vi "环境数据发送帧.vi"(10 "环境变量":T1, 11 "用户地址":string) -> (2 "报文长度":i32, 3 "字符串":string)   [LabVIEW 2016, in "环境动力监测库.lvlib" / "NMEA.lvlib"]
uses:
  NMEA.lvlib
panel:
  out "data":T2 {"数据类别" items=["水样数据"=0, "标样数据"=1, "零点核查数据"=2, "跨度核查数据"=3, "环境变量"=4, "水样数据补传"=16, "标样核查数据补传"=17, "零点核查数据补传"=18, "跨度核查数据补传"=19]; "数组"."污染物" items=["水温"=1, "浊度"=2, "DO"=3, "pH"=4, "ORP"=5, "比电导率"=6, "叶绿素a"=7, "氨氮"=8, "亚硝氮"=9, "硫化物"=10, "电压"=11, "温度"=12, "湿度"=13, "GPS经度"=14, "GPS纬度"=15, "BD经度"=16, "BD纬度"=17]; "数组"."标识" items=["N"=1, "T"=2, "L"=3, "D"=4, "Z"=5, "M"=6, "hd"=7]}
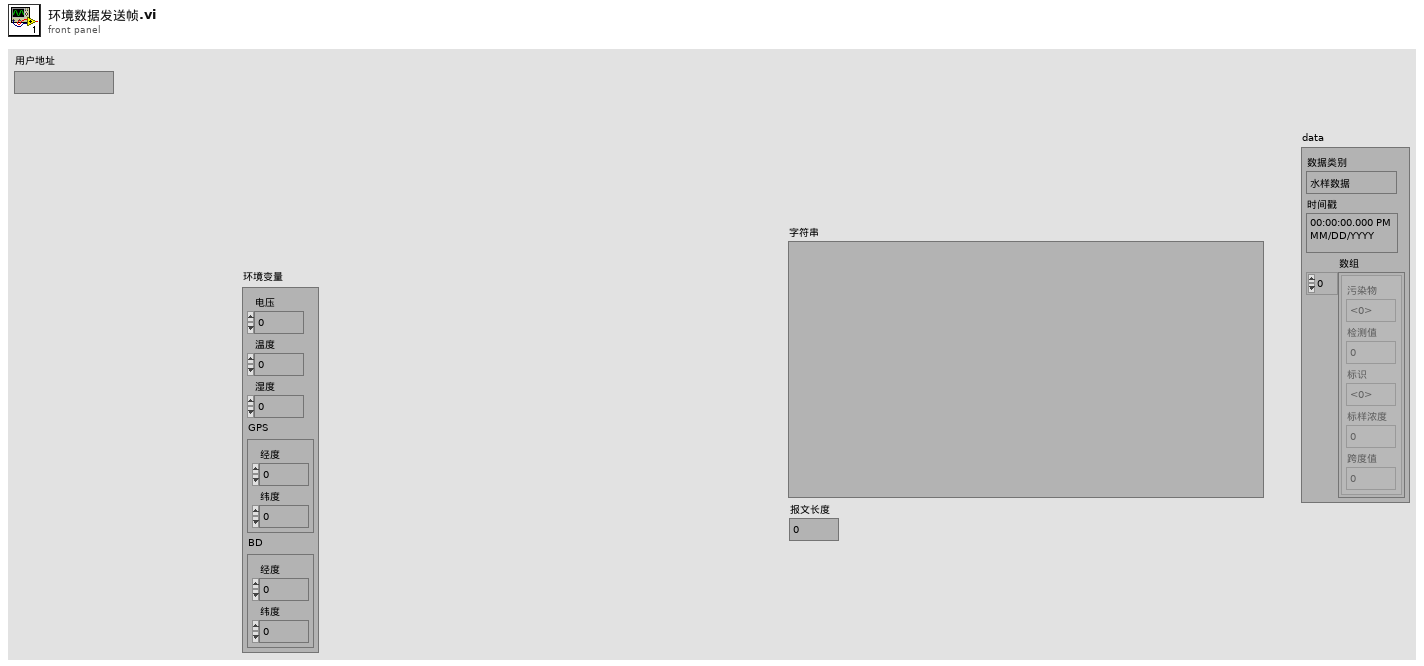
[diagram p1: front panel]
types:
  T1 = cluster{"电压":dbl, "温度":dbl, "湿度":dbl, "GPS":cluster{"经度":dbl, "纬度":dbl}, "BD":cluster{"经度":dbl, "纬度":dbl}}
  T2 = cluster{"数据类别":u16, "时间戳":timestamp, "数组":cluster{"污染物":u16, "检测值":dbl, "标识":u16, "标样浓度":dbl, "跨度值":dbl}[]}
  T3 = cluster{"污染物":u16, "检测值":dbl, "标识":u16, "标样浓度":dbl, "跨度值":dbl}
  T4 = cluster{"污染物":u16, "检测值":dbl, "标识":u16, "标样浓度":dbl, "跨度值":dbl}[]
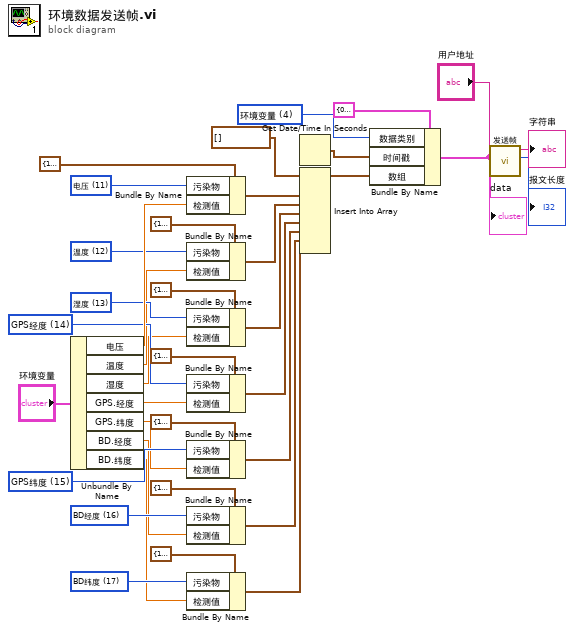
[diagram p0: block diagram]
diagram:
  w14 = u16 17 items=["水温"=1, "浊度"=2, "DO"=3, "pH"=4, "ORP"=5, "比电导率"=6, "叶绿素a"=7, "氨氮"=8, "亚硝氮"=9, "硫化物"=10, "电压"=11, "温度"=12, "湿度"=13, "GPS经度"=14, "GPS纬度"=15, "BD经度"=16, "BD纬度"=17] ("污染物")
  w15 = u16 16 items=["水温"=1, "浊度"=2, "DO"=3, "pH"=4, "ORP"=5, "比电导率"=6, "叶绿素a"=7, "氨氮"=8, "亚硝氮"=9, "硫化物"=10, "电压"=11, "温度"=12, "湿度"=13, "GPS经度"=14, "GPS纬度"=15, "BD经度"=16, "BD纬度"=17] ("污染物")
  w18 = u16 15 items=["水温"=1, "浊度"=2, "DO"=3, "pH"=4, "ORP"=5, "比电导率"=6, "叶绿素a"=7, "氨氮"=8, "亚硝氮"=9, "硫化物"=10, "电压"=11, "温度"=12, "湿度"=13, "GPS经度"=14, "GPS纬度"=15, "BD经度"=16, "BD纬度"=17] ("污染物")
  w19 = u16 14 items=["水温"=1, "浊度"=2, "DO"=3, "pH"=4, "ORP"=5, "比电导率"=6, "叶绿素a"=7, "氨氮"=8, "亚硝氮"=9, "硫化物"=10, "电压"=11, "温度"=12, "湿度"=13, "GPS经度"=14, "GPS纬度"=15, "BD经度"=16, "BD纬度"=17] ("污染物")
  w22 = u16 13 items=["水温"=1, "浊度"=2, "DO"=3, "pH"=4, "ORP"=5, "比电导率"=6, "叶绿素a"=7, "氨氮"=8, "亚硝氮"=9, "硫化物"=10, "电压"=11, "温度"=12, "湿度"=13, "GPS经度"=14, "GPS纬度"=15, "BD经度"=16, "BD纬度"=17] ("污染物")
  w23 = u16 12 items=["水温"=1, "浊度"=2, "DO"=3, "pH"=4, "ORP"=5, "比电导率"=6, "叶绿素a"=7, "氨氮"=8, "亚硝氮"=9, "硫化物"=10, "电压"=11, "温度"=12, "湿度"=13, "GPS经度"=14, "GPS纬度"=15, "BD经度"=16, "BD纬度"=17] ("污染物")
  w26 = u16 11 items=["水温"=1, "浊度"=2, "DO"=3, "pH"=4, "ORP"=5, "比电导率"=6, "叶绿素a"=7, "氨氮"=8, "亚硝氮"=9, "硫化物"=10, "电压"=11, "温度"=12, "湿度"=13, "GPS经度"=14, "GPS纬度"=15, "BD经度"=16, "BD纬度"=17] ("污染物")
  w30 = u16 4 items=["水样数据"=0, "标样数据"=1, "零点核查数据"=2, "跨度核查数据"=3, "环境变量"=4, "水样数据补传"=16, "标样核查数据补传"=17, "零点核查数据补传"=18, "跨度核查数据补传"=19] ("数据类别")
  n1 = Unbundle By Name("环境变量") -> ("电压"=w25:dbl, "温度"=w6:dbl, "湿度"=w5:dbl, "GPS.经度"=w4:dbl, "GPS.纬度"=w3:dbl, "BD.经度"=w2:dbl, "BD.纬度"=w1:dbl)
  n2 = Bundle By Name(cluster=T3 {"污染物"=11, "检测值"=0.0, "标识"=0, "标样浓度"=0.0, "跨度值"=0.0} ("数据"), "污染物"=w26, "检测值"=w25) -> (w34:T3)
  n3 = Bundle By Name(cluster=T3 {"污染物"=11, "检测值"=0.0, "标识"=0, "标样浓度"=0.0, "跨度值"=0.0} ("数据"), "污染物"=w23, "检测值"=w6) -> (w12:T3)
  n4 = Bundle By Name(cluster=T3 {"污染物"=11, "检测值"=0.0, "标识"=0, "标样浓度"=0.0, "跨度值"=0.0} ("数据"), "污染物"=w22, "检测值"=w5) -> (w11:T3)
  n5 = Bundle By Name(cluster=T3 {"污染物"=11, "检测值"=0.0, "标识"=0, "标样浓度"=0.0, "跨度值"=0.0} ("数据"), "污染物"=w19, "检测值"=w4) -> (w10:T3)
  n6 = Bundle By Name(cluster=T3 {"污染物"=11, "检测值"=0.0, "标识"=0, "标样浓度"=0.0, "跨度值"=0.0} ("数据"), "污染物"=w18, "检测值"=w3) -> (w9:T3)
  n7 = Bundle By Name(cluster=T3 {"污染物"=11, "检测值"=0.0, "标识"=0, "标样浓度"=0.0, "跨度值"=0.0} ("数据"), "污染物"=w15, "检测值"=w2) -> (w8:T3)
  n8 = Bundle By Name(cluster=T3 {"污染物"=11, "检测值"=0.0, "标识"=0, "标样浓度"=0.0, "跨度值"=0.0} ("数据"), "污染物"=w14, "检测值"=w1) -> (w7:T3)
  n9 = Get Date/Time In Seconds() -> (seconds since 1Jan1904=w33:timestamp)
  n10 = Insert Into Array(array=T4 [] ("数组"), new element #1=w34, new element #2=w12, new element #3=w11, new element #4=w10, new element #5=w9, new element #6=w8, new element #7=w7) -> (w27:T4)  [unwired: 1 in]
  n11 = Bundle By Name(cluster=T2 {"数据类别"=0, "时间戳"=timestamp(0 s since 1904-01-01), "数组"=[]} ("data"), "数据类别"=w30, "时间戳"=w33, "数组"=w27) -> (w29:T2)
  "data" <- w29
  n12 = call "发送帧.vi"("data"=w29, "用户地址"="用户地址") -> ("报文长度"=→"报文长度":i32, "字符串"=→"字符串":string)  [unwired: 8 in]
